vi "whatsVisibleTI.vi"(11 "UplotInfoArray":T1(array[cluster])) -> (1 "Targets Visible":bool[](array[boolean]))   [LabVIEW 2013]
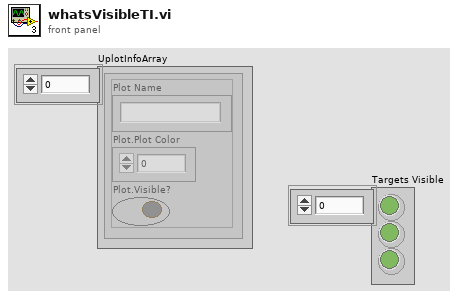
[diagram p1: front panel]
types:
  T1 = cluster{"Plot Name":string, "Plot.Plot Color":u32, "Plot.Visible?":bool}[]
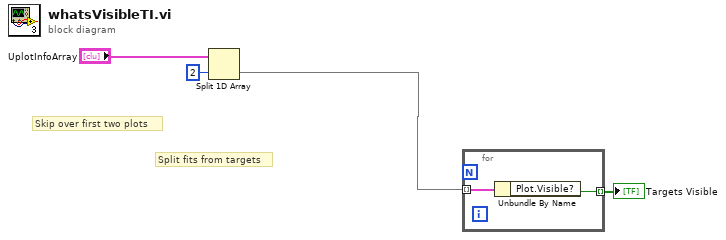
[diagram p0: block diagram]
diagram:
  # "Split fits from targets"
  # "Skip over first two plots"
  n1 = Split 1D Array(array="UplotInfoArray", index=2) -> (second subarray=w1:T1)  [unwired: 1 out]
  n2 = for {
    tunnel: w1 -> [w6] mode=indexing
    tunnel: [w5] -> w2 mode=indexing
    n3 = Unbundle By Name(w6) -> ("Plot.Visible?"=w5:bool)
  }
  "Targets Visible" <- w2
